vi "LM235_Conv.vi"() -> ()   [LabVIEW 2025]
panel:
  in  "Div":dbl=1.0
  out "C":dbl format="%#_6f"
  in  "V":dbl
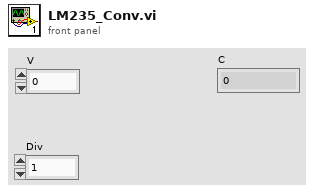
[diagram p1: front panel]
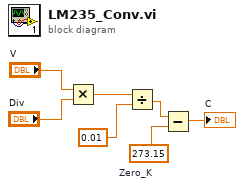
[diagram p0: block diagram]
diagram:
  w5 = 273.15  # Zero_K
  n1 = Multiply(x="V", y="Div") -> (x*y=w3:dbl)
  n2 = Divide(x=w3, y=0.01) -> (x/y=w2:dbl)
  n3 = Subtract(x=w2, y=w5) -> (x-y=→"C":dbl)
